vi "Cal_angle_order.vi"(7 "Deg/pixels?":bool, 8 "Thickness":dbl=210.0 format="%.3f", 9 "Wavelength":dbl=1.21 format="%.3f", 10 "Angle 2 (deg)":dbl=8.5 format="%.3f", 11 "Angle 1  (deg)":dbl=2.0 format="%.3f") -> (1 "dOrder":dbl=-1.0193819817582153 format="%.3f", 2 "Order 2":dbl=1218.6278126663108 format="%.3f", 3 "Order 1":dbl=1219.647194648069 format="%.3f")   [LabVIEW 2010]
panel:
  in  "refr inx master from":dbl=3.513918800819122
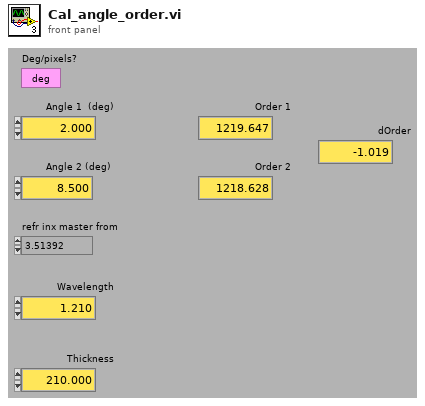
[diagram p1: front panel]
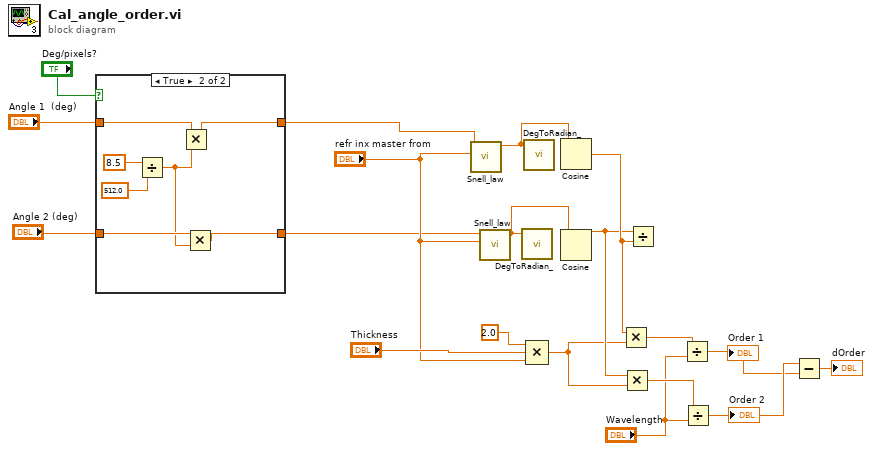
[diagram p0: block diagram]
diagram:
  n1 = case shown="True" "Deg/pixels?" {
    tunnel: [w21 w23] -> w5
    tunnel: [w20 w24] -> w4
    tunnel: "Angle 1  (deg)" -> [w21 w26]
    tunnel: "Angle 2 (deg)" -> [w20 w25]
    frame False {
    }
    frame True {
      n2 = Divide(x=8.5, y=512.0 ("x")) -> (x/y=w22:dbl)
      n3 = Multiply(x=w26, y=w22) -> (x*y=w23:dbl)
      n4 = Multiply(x=w25, y=w22) -> (x*y=w24:dbl)
    }
  }
  n5 = call "Snell_law.vi"("Refr index"="refr inx master from", "Angle in ext (deg)"=w5) -> ("Angle out int (rad)"=w18:dbl)  [unwired: 8 in, 1 out]
  n6 = call "Snell_law.vi"("Refr index"="refr inx master from", "Angle in ext (deg)"=w4) -> ("Angle out int (rad)"=w19:dbl)  [unwired: 8 in, 1 out]
  n7 = call "DegToRadian_.vi"("Angle deg"=w19) -> ()  [unwired: 4 in, 1 out]
  n8 = call "DegToRadian_.vi"("Angle deg"=w18) -> ()  [unwired: 4 in, 1 out]
  n9 = Compound Arithmetic op=MULTIPLY(2.0 ("value"), "Thickness", "refr inx master from") -> (w12:dbl)
  n10 = Cosine(x=w18) -> (cos(x)=w14:dbl)
  n11 = Cosine(x=w19) -> (cos(x)=w13:dbl)
  n12 = Multiply(x=w14, y=w12) -> (x*y=w11:dbl)
  n13 = Multiply(x=w13, y=w12) -> (x*y=w10:dbl)
  n14 = Divide(x=w13, y=w14) -> ()  [unwired: 1 out]
  n15 = Divide(x=w11, y="Wavelength") -> (x/y=w7:dbl)
  "Order 1" <- w7
  n16 = Divide(x=w10, y="Wavelength") -> (x/y=w8:dbl)
  "Order 2" <- w8
  n17 = Subtract(x=w8, y=w7) -> (x-y=→"dOrder":dbl)
